vi "ProdaNG.Configurator.Popup.Edit.vi"(6 "units simple":T1[](array[typedef]), 9 "Selected elements values":T2[](array[typedef]), 10 "Elements to edit":T3[](array[typedef])) -> (1 "Selected elements values out":T2[](array[typedef]), 4 "Reason out":string, 5 "OK?":bool)   [LabVIEW 2016]
uses:
  ProdaNG.Tree.Fglb.Data.ctl
  ProdaNG.Tree.Fglb.Element.ctl
  ProdaNG.Tree.Fglb.Value.ctl
  Controls/ProdaNG.UnitSimple.ctl
panel:
  in  "Unit":i32(ring) items=[""=0, "unknown"=-1, "%"=1, "bar"=2, "bar (abs)"=3, "mbar"=4, "bar/s"=5, "mbar/s"=6, "l/min"=7, "s"=8, "ms"=9, "mm"=10, "N"=11, "A"=12, "V"=13, "ohm"=14, "kohm"=15, "Hz"=16, "angle"=17, "count"=18, "bool"=19, "ASCII"=20, "Nm"=21, "kg"=22, "obr/min"=23, "ccm/min"=24, "mA"=25, "digit"=26, "us"=27, "stC"=28, "mBar/s"=29, "mA/s"=30, "undefined"=31, "WGrad"=32, "mH"=33, "-"=34, "tics"=35, "Nr"=36, "bar/min"=37, "us/mm"=38, "deg"=39, "mbar/deg"=40, "deg/s"=41]
  in  "Value2":dbl caption="High Limit" format="%.3f"
  in  "Value1":dbl caption="Low Limit / Param Value" format="%.3f"
  in  "Order":i32
  in  "Reason":string
  in  "Description":string
  in  "Button.Cancel":bool
  in  "Button.OK":bool
  out "Msg":string
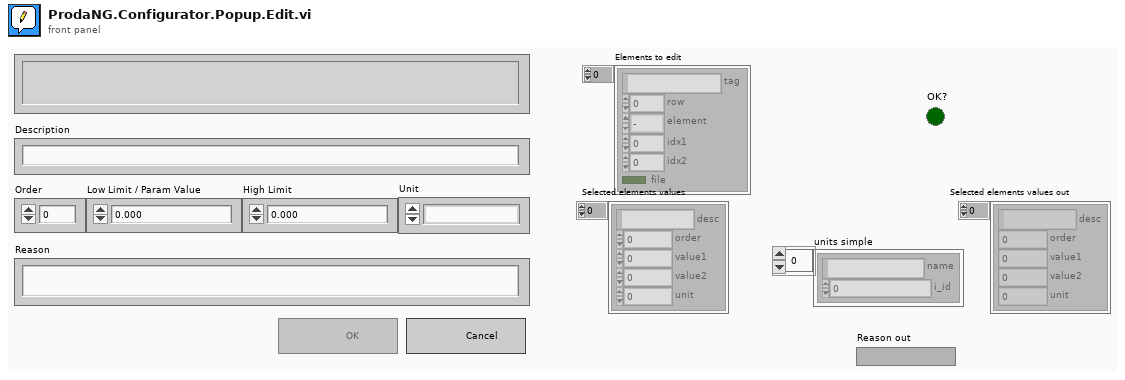
[diagram p1: front panel]
types:
  T1 = typedef "ProdaNG.UnitSimple.ctl" = cluster{"name":string, "i_id":i32}
  T2 = typedef "ProdaNG.Tree.Fglb.Value.ctl" = cluster{"desc":string, "order":i32, "value1":dbl, "value2":dbl, "unit":i32}
  T3 = typedef "ProdaNG.Tree.Fglb.Data.ctl" = cluster{"tag":string, "row":i32, "element":T4, "idx1":i32, "idx2":i32, "file":bool}
  T4 = typedef "ProdaNG.Tree.Fglb.Element.ctl" = enum16{"-", "PP", "TS", "TP", "TV"}
  T5 = enum8{"Enabled", "Disabled", "Disabled and Grayed Out"}
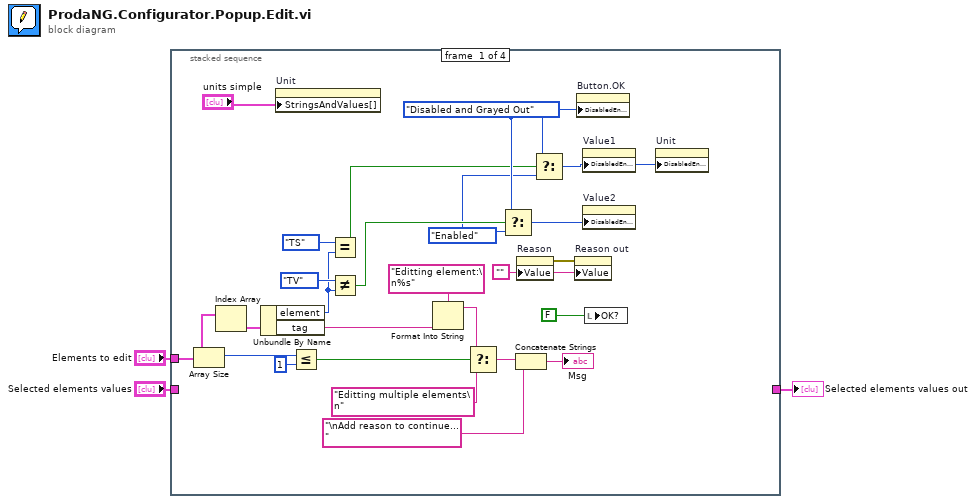
[diagram p0: block diagram]
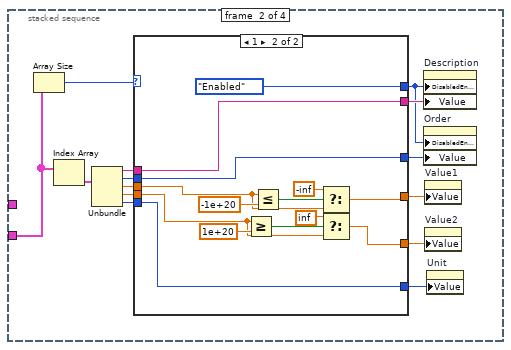
[diagram p2: hidden frame]
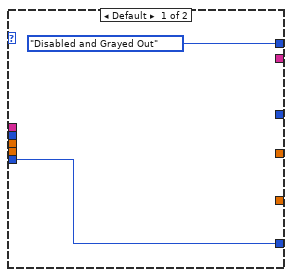
[diagram p3: hidden frame]
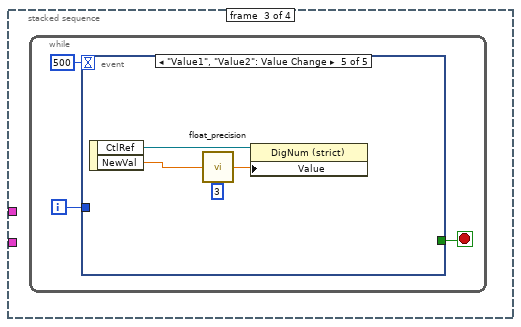
[diagram p4: hidden frame]
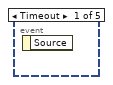
[diagram p5: hidden frame]
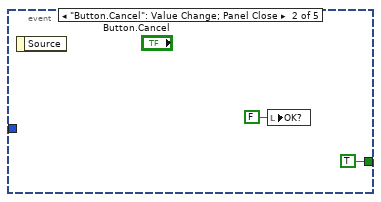
[diagram p6: hidden frame]
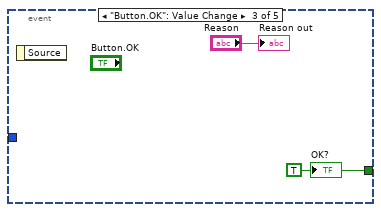
[diagram p7: hidden frame]
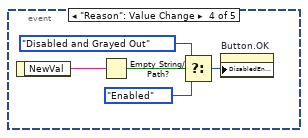
[diagram p8: hidden frame]
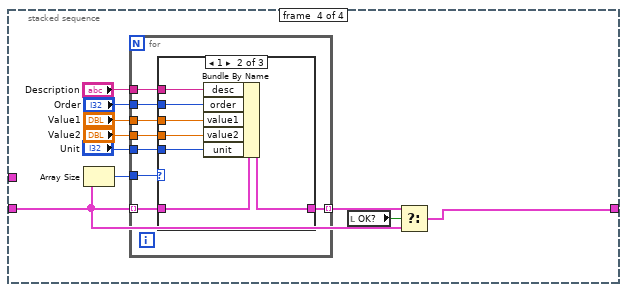
[diagram p9: hidden frame]
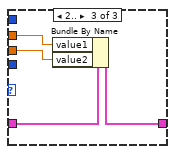
[diagram p11: hidden frame]
diagram:
  n1 = stacked-sequence {
    tunnel: "Elements to edit" -> [w24 _ _ _]
    tunnel: "Selected elements values" -> [_ w42 _ w77]
    tunnel: [_ _ _ w76] -> w1
    frame #0 {
      w5 = T5."Enabled" ("Disabled")
      w14 = ""
      w7 = T5."Disabled and Grayed Out" ("Disabled")
      n2 = Array Size(array=w24) -> (size(s)=w27:i32)
      n3 = Index Array(array=w24) -> (element=w23:T3)  [unwired: 1 in]
      n4 = Unbundle By Name(w23) -> ("element"=w9:T4, "tag"=w22:string)
      n5 = property on="Unit" class="Ring (strict)"("StringsAndValues[]"="units simple") -> ()  [unwired: 2 in, 2 out]
      n6 = Less Or Equal?(x=w27, y=1) -> (x <= y?=w25:bool)
      n7 = Equal?(x=ProdaNG.Tree.Fglb.Element."TS", y=w9) -> (x = y?=w6:bool)
      n8 = Not Equal?(x=ProdaNG.Tree.Fglb.Element."TV", y=w9) -> (x != y?=w11:bool)
      n9 = Format Into String(format string="Editting element:\n%s", w22) -> (resulting string=w20:string)  [unwired: 2 in, 1 out]
      n10 = Select(t=w20, s=w25, f="Editting multiple elements\n" ("format string")) -> (s? t:f=w18:string)
      n11 = Select(t=w7, s=w11, f=w5) -> (s? t:f=w10:T5)
      n12 = Concatenate Strings(w18, "\nAdd reason to continue..." ("Msg")) -> (→"Msg":string)
      n13 = property on="Reason" class="Str"("Value"=w14) -> (error out=w15:errorcluster)  [unwired: 2 in, 1 out]
      n14 = Select(t=w7, s=w6, f=w5) -> (s? t:f=w4:T5)
      n15 = property on="Reason out" class="Str"(error in=w15, "Value"=w14) -> ()  [unwired: 1 in, 2 out]
      n16 = property on="Button.OK" class="Bool"("DisabledEnum"=w7) -> ()  [unwired: 2 in, 2 out]
      n17 = property on="Value1" class="DigNum (strict)"("DisabledEnum"=w4) -> ()  [unwired: 2 in, 2 out]
      n18 = property on="Value2" class="DigNum (strict)"("DisabledEnum"=w10) -> ()  [unwired: 2 in, 2 out]
      n19 = local write "OK?"(FALSE ("OK?")) -> ()
      n20 = property on="Unit" class="Ring (strict)"("DisabledEnum"=w4) -> ()  [unwired: 2 in, 2 out]
    }
    frame #1 {
      n21 = Array Size(array=w42) -> (size(s)=w40:i32)
      n22 = Index Array(array=w42) -> (element=w41:T2)  [unwired: 1 in]
      n23 = Unbundle(w41) -> ("desc"=w38:string, "order"=w37:i32, "value1"=w34:dbl, "value2"=w33:dbl, "unit"=w29:i32)
      n24 = case shown="1" w40 {
        tunnel: [T5."Disabled and Grayed Out" ("Disabled") T5."Enabled" ("Disabled")] -> w35
        tunnel: [_ w57] -> w39
        tunnel: w38 -> [_ w57]
        tunnel: w37 -> [_ w56]
        tunnel: [_ w56] -> w36
        tunnel: w34 -> [_ w46]
        tunnel: w33 -> [_ w47]
        tunnel: [_ w49] -> w32
        tunnel: [_ w48] -> w31
        tunnel: [w43 w45] -> w30
        tunnel: w29 -> [w43 w45]
        frame Default {
        }
        frame 1 {
          n25 = Greater Or Equal?(x=w47, y=1e+20) -> (x >= y?=w54:bool)
          n26 = Less Or Equal?(x=w46, y=-1e+20) -> (x <= y?=w55:bool)
          n27 = Select(t=-inf, s=w55, f=w46) -> (s? t:f=w49:dbl)
          n28 = Select(t=inf, s=w54, f=w47) -> (s? t:f=w48:dbl)
        }
      }
      n29 = property on="Description" class="Str"("DisabledEnum"=w35, "Value"=w39) -> ()  [unwired: 2 in, 2 out]
      n30 = property on="Order" class="DigNum (strict)"("DisabledEnum"=w35, "Value"=w36) -> ()  [unwired: 2 in, 2 out]
      n31 = property on="Value1" class="DigNum (strict)"("Value"=w32) -> ()  [unwired: 2 in, 2 out]
      n32 = property on="Value2" class="DigNum (strict)"("Value"=w31) -> ()  [unwired: 2 in, 2 out]
      n33 = property on="Unit" class="Ring (strict)"("Value"=w30) -> ()  [unwired: 2 in, 2 out]
    }
    frame #2 {
      n34 = while {
        i -> [w59]
        stop <- w61 stop-if-true
        n35 = event shown="[4] \"Value1\", \"Value2\": Value Change" {
          selector: _ -> [_ _ _ _ _]
          dyn-events: _ -> [_ _ _ _ _]
          timeout: 500 -> [_ _ _ _ _]
          tunnel: [_ TRUE ("OK?") w65 _ _] -> w61
          tunnel: w59 -> [_ _ _ _ _]
          event Timeout {
            n36 = event-data() -> ()  [unwired: 1 in, 1 out]
          }
          event "Button.Cancel": Value Change; Panel Close {
            n37 = event-data() -> ()  [unwired: 1 in, 1 out]
            n38 = local write "OK?"(FALSE ("OK?")) -> ()
          }
          event "Button.OK": Value Change {
            w65 = TRUE ("OK?")
            n39 = event-data() -> ()  [unwired: 1 in, 1 out]
            "OK?" <- w65
            "Reason out" <- "Reason"
          }
          event "Reason": Value Change {
            n40 = event-data() -> ("NewVal"=w66:string)  [unwired: 1 in]
            n41 = Empty String/Path?(string/path=w66) -> (empty?=w70:bool)
            n42 = Select(t=T5."Disabled and Grayed Out" ("Disabled"), s=w70, f=T5."Enabled" ("Disabled")) -> (s? t:f=w67:T5)
            n43 = property on="Button.OK" class="Bool"("DisabledEnum"=w67) -> ()  [unwired: 2 in, 2 out]
          }
          event "Value1", "Value2": Value Change {
            n44 = event-data() -> ("CtlRef"=w72:refnum<vi>, "NewVal"=w73:dbl)  [unwired: 1 in]
            n45 = call "float_precision.vi"("input"=w73, "precision"=3) -> ("output"=w71:dbl)
            n46 = property class="DigNum (strict)"(reference=w72, "Value"=w71) -> ()  [unwired: 1 in, 2 out]
          }
        }
      }
    }
    frame #3 {
      n47 = Array Size(array=w77) -> (size(s)=w84:i32)
      n48 = for {
        tunnel: w77 -> [w90] mode=indexing
        tunnel: w84 -> [w92]
        tunnel: "Value2" -> [w91]
        tunnel: "Value1" -> [w89]
        tunnel: "Order" -> [w88]
        tunnel: "Description" -> [w87]
        tunnel: [w86] -> w78 mode=indexing
        tunnel: "Unit" -> [w85]
        n49 = case shown="1" w92 {
          tunnel: w91 -> [_ w99 w103]
          tunnel: w90 -> [w93 w96 w104]
          tunnel: w89 -> [_ w100 w102]
          tunnel: w88 -> [_ w98 _]
          tunnel: w87 -> [_ w97 _]
          tunnel: [w93 w95 w101] -> w86
          tunnel: w85 -> [_ w94 _]
          frame Default {
          }
          frame 1 {
            n50 = Bundle By Name(cluster=w96, "desc"=w97, "order"=w98, "value1"=w100, "value2"=w99, "unit"=w94) -> (w95:T2)
          }
          frame 2.. {
            n51 = Bundle By Name(cluster=w104, "value1"=w102, "value2"=w103) -> (w101:T2)
          }
        }
      }
      n52 = local read "OK?"() -> (w79:bool)
      n53 = Select(t=w78, s=w79, f=w77) -> (s? t:f=w76:T2[])
    }
  }
  "Selected elements values out" <- w1
